vi "Command Finished.vi"(8 "error in (no error)":errorcluster, 11 "Running Command in":refnum<class "Running Command.lvclass">) -> (0 "error out":errorcluster, 3 "Running Command out":refnum<class "Running Command.lvclass">)   [LabVIEW 2013, in "Robot Actors.lvlib" / "Command Processor.lvlib" / "Running Command.lvclass"]
uses:
  Running Command.lvclass
  Command Processor Class/Command Processor.lvclass
  <vilib>/ActorFramework/Actor/Actor.lvclass/Actor.ctl
  <vilib>/ActorFramework/Message Enqueuer/Message Enqueuer.lvclass/Message Enqueuer.ctl
  <vilib>/ActorFramework/Message Enqueuer/Init from Existing Queue.vi
  <vilib>/ActorFramework/Message Enqueuer/Enqueue.vi
  <vilib>/ActorFramework/Message Priority Queue/Priority Enqueue.vi
  <vilib>/ActorFramework/Message Enqueuer/Message Enqueuer.lvclass
  Command Processor Messages/Go To No Command Msg/Go To No Command Msg.lvclass
  <vilib>/ActorFramework/Actor/Actor.lvclass
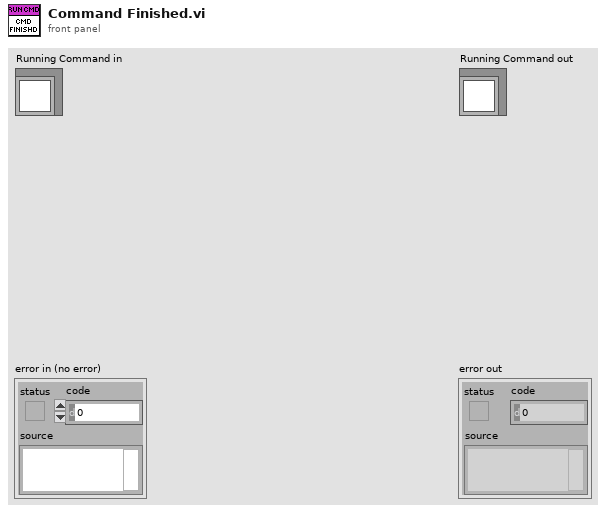
[diagram p1: front panel]
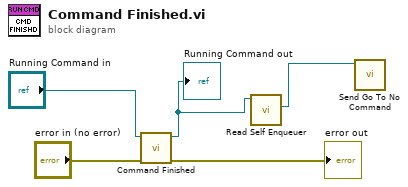
[diagram p0: block diagram]
diagram:
  n1 = call-parent "Command Finished.vi"("error in (no error)"="error in (no error)", "Command Processor in"="Running Command in") -> ("error out"=→"error out":errorcluster, "Command Processor out"=w2:refnum<class "Running Command.lvclass">)  [unwired: 8 in]
  "Running Command out" <- w2
  n2 = call <vilib>:"Read Self Enqueuer.vi"("Actor"=w2) -> ("Self Enqueuer"=w1:refnum<class "Message Enqueuer.lvclass">)  [unwired: 10 in]
  n3 = call "Send Go To No Command.vi"("Message Enqueuer"=w1) -> ()  [unwired: 9 in, 2 out]
